vi "Read Configuration Items.vi"(8 "error in":errorcluster, 11 "Base Software in":refnum<class "Main.lvclass">) -> (0 "error out":errorcluster, 3 "Base Software out":refnum<class "Main.lvclass">)   [LabVIEW 2023, in "Main.lvlib" / "Main.lvclass"]
uses:
  Project/Main.lvclass
  C:/Users/Public/Documents/Development/builds/Engine/Engine.lvlibp/Project/Engine.lvclass
  builds/Tools/Config.lvlibp/Config.lvclass
  Project/Main.lvclass/Main.ctl
  builds/Engine/Engine.lvlibp/Accessors/Read Directory.vi
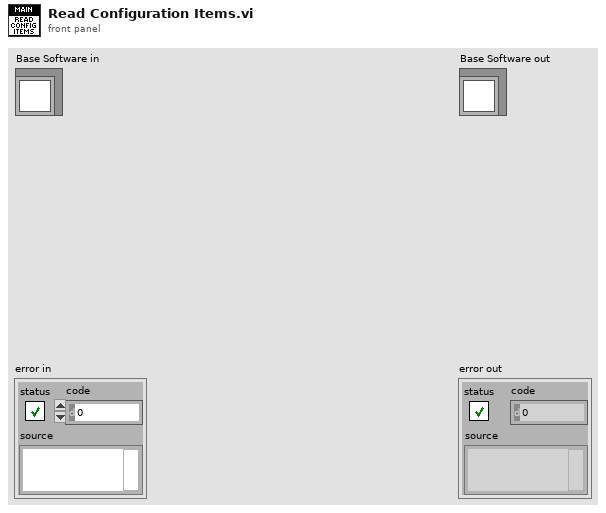
[diagram p1: front panel]
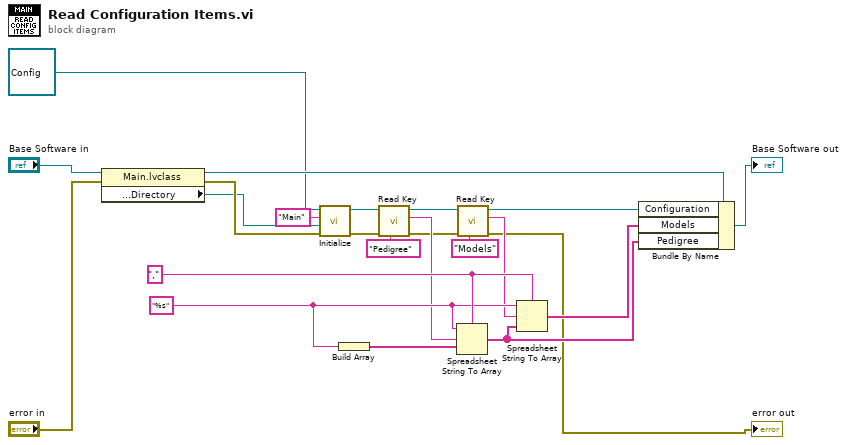
[diagram p0: block diagram]
diagram:
  w23 = "," ("delimiter (Tab)")
  w20 = "%s" ("format string")
  n1 = property class="Main.lvclass"(reference="Base Software in", error in="error in") -> (reference out=w6:refnum<class "Main.lvclass">, error out=w13:errorcluster, "Accessors:Application:Information:Directory"=w12:path)
  n2 = call-dynamic "Initialize.vi"("error in"=w13, "Path"=w12, "Device"="Main", "Config in"=refnum<class "Config.lvclass"> refnum) -> ("error out"=w7:errorcluster, "Config out"=w8:refnum<class "Config.lvclass">)  [unwired: 6 in]
  n3 = Build Array(w20) -> (w21:string[])
  n4 = call "Read Key.vi"("Key Name"="Pedigree", "error in"=w7, "Config in"=w8) -> ("error out"=w10:errorcluster, "Key Value"=w18:string, "Config out"=w9:refnum<class "Config.lvclass">)  [unwired: 6 in]
  n5 = Spreadsheet String To Array(delimiter (Tab)=w23, format string=w20, spreadsheet string=w18, array type (2D Dbl)=w21) -> (array=w22:string[])
  n6 = call "Read Key.vi"("Key Name"="Models", "error in"=w10, "Config in"=w9) -> ("error out"=→"error out":errorcluster, "Key Value"=w17:string, "Config out"=w11:refnum<class "Config.lvclass">)  [unwired: 6 in]
  n7 = Spreadsheet String To Array(delimiter (Tab)=w23, format string=w20, spreadsheet string=w17, array type (2D Dbl)=w22) -> (array=w19:string[])
  n8 = Bundle By Name(cluster=w6, "Configuration"=w11, "Models"=w19, "Pedigree"=w22) -> (→"Base Software out":refnum<class "Main.lvclass">)
